vi "PID water height and temperature.vi"(4 "State":i16, 5 "Time":dbl format="%.2f", 6 "Sensor Values":dbl[](array[numeric]), 7 "Set Points":dbl[](array[numeric])) -> (0 "required data":T1={"Set Point names"=["cold/hot output (0/1)", "valve on time (s)", "T target (C)", "H min (cm)", "H abort fill (cm)", "P Kc", "I Ti (s)", "D Td (s)"], "required number of setpoints"=8, "required number of sensors"=2, "Sensor names"=["temperature (C)", "water depth (cm)"]}, 3 "output value":dbl)   [LabVIEW 2019]
uses:
  <vilib>/addons/control/pid/pid.llb/PID (DBL).vi
  <vilib>/addons/control/pid/NI_PID_pid.lvlib
panel:
  out "PID":dbl
  out "Enum 2":enum16{"Waiting", "Filling"}(ring)
  # "Enter the correct information for this control code in the required data structure below. Then make the current value default by right clicking on the border of the data structure."
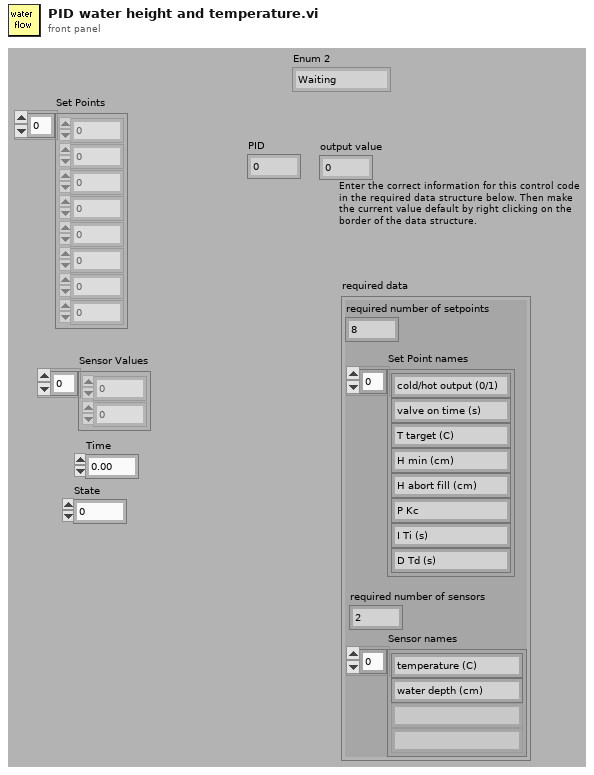
[diagram p1: front panel]
types:
  T1 = cluster{"Set Point names":string[], "required number of setpoints":u8, "required number of sensors":u8, "Sensor names":string[]}
  T2 = cluster{"Set Points[0]":dbl, "Set Points[1]":dbl, "Set Points[2]":dbl, "Set Points[3]":dbl, "Set Points[4]":dbl, "Set Points[5]":dbl, "Set Points[6]":dbl, "Set Points[7]":dbl}
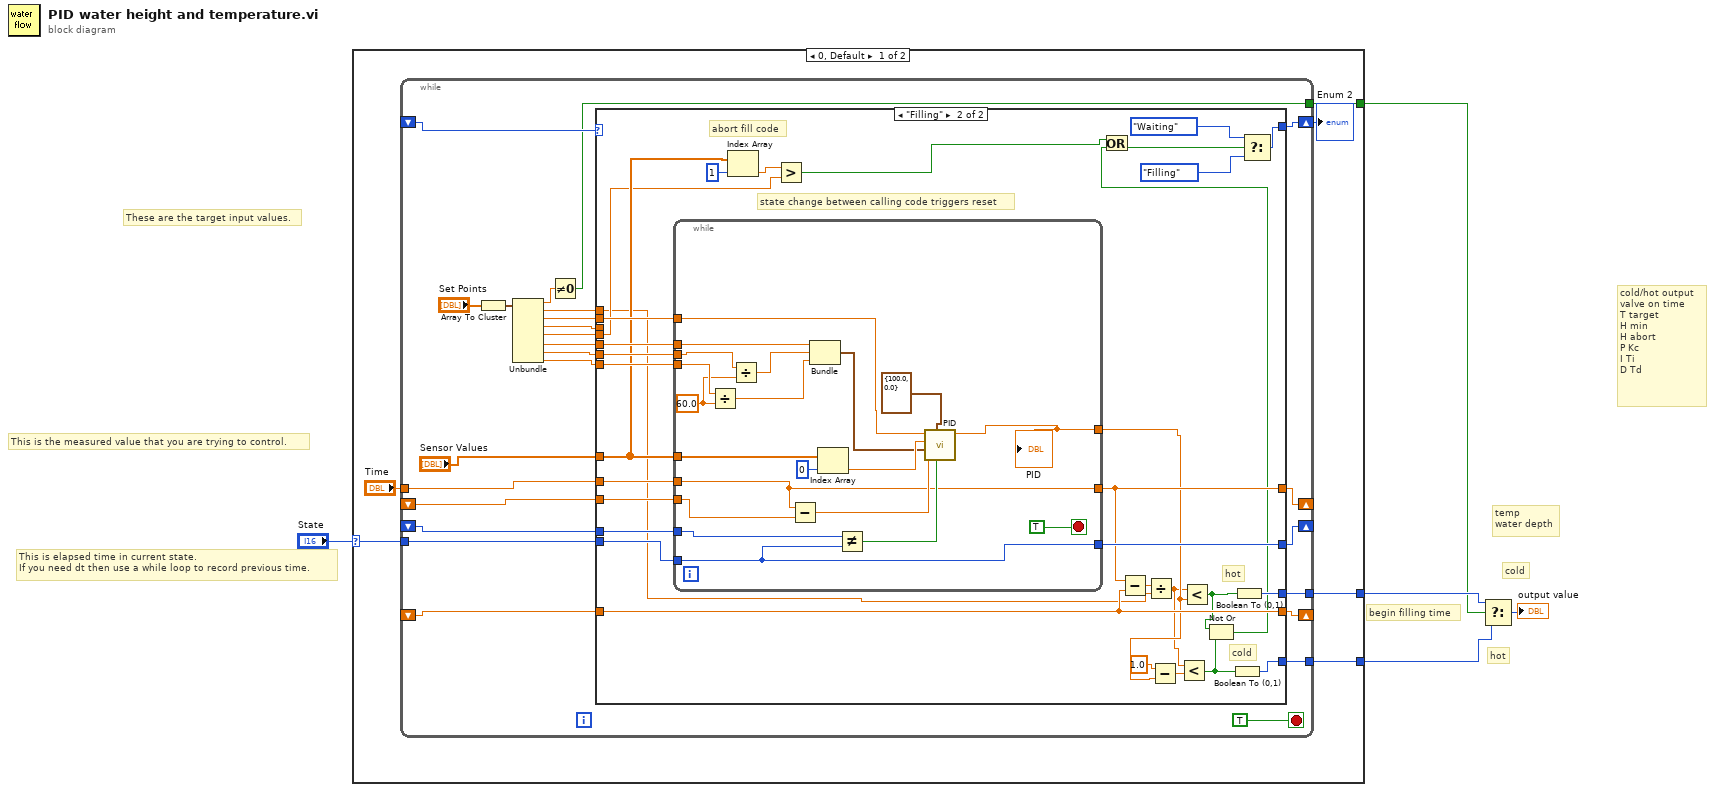
[diagram p0: block diagram]
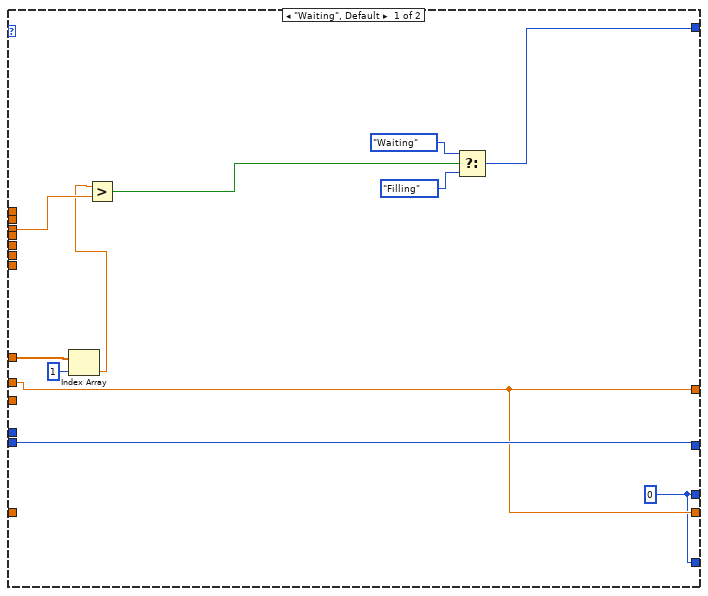
[diagram p2: hidden frame]
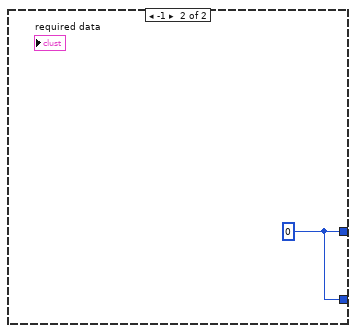
[diagram p3: hidden frame]
diagram:
  # "begin filling time"
  # "hot"
  # "cold"
  # "temp\nwater depth"
  # "cold/hot output\nvalve on time\nT target\nH min\nH abort\nP Kc\nI Ti\nD Td"
  # "These are the target input values."
  # "This is the measured value that you are trying to control."
  # "This is elapsed time in current state.\nIf you need dt then use a while loop to record previous time."
  n1 = case shown="0, Default" "State" {
    selector: "State" -> [w11 _]
    tunnel: [w9 _] -> w2
    tunnel: [w8 w99] -> w3
    tunnel: [w7 w99] -> w1
    frame 0, Default {
      n2 = while {
        tunnel: w11 -> [w36]
        shift-right: [w34] -> w6
        shift-left: _ -> [w24]
        shift-right: [w21] -> _
        shift-left: _ -> [w22]
        shift-right: [w18] -> _
        shift-left: _ -> [w20]
        tunnel: "Time" -> [w19]
        tunnel: [w16] -> w9
        shift-right: [w15] -> _
        shift-left: _ -> [w14]
        tunnel: [w13] -> w8
        tunnel: [w12] -> w7
        stop <- TRUE stop-if-true
        n3 = Array To Cluster(array="Set Points") -> (cluster=w32:T2)
        n4 = Unbundle(w32) -> ("Set Points[0]"=w17:dbl, "Set Points[1]"=w26:dbl, "Set Points[2]"=w27:dbl, "Set Points[3]"=w25:dbl, "Set Points[4]"=w23:dbl, "Set Points[5]"=w30:dbl, "Set Points[6]"=w29:dbl, "Set Points[7]"=w28:dbl)
        n5 = Not Equal To 0?(x=w17) -> (x != 0?=w16:bool)
        n6 = case shown="\"Filling\"" w24 {
          tunnel: w36 -> [w39 w78]
          tunnel: [w45 w70] -> w34
          tunnel: "Sensor Values" -> [w43 w68]
          tunnel: w30 -> [_ w77]
          tunnel: w29 -> [_ w76]
          tunnel: w28 -> [_ w75]
          tunnel: w27 -> [_ w74]
          tunnel: w26 -> [_ w59]
          tunnel: w25 -> [w42 _]
          tunnel: w20 -> [_ w73]
          tunnel: w23 -> [_ w66]
          tunnel: w22 -> [_ w65]
          tunnel: [w39 w64] -> w21
          tunnel: w19 -> [w38 w63]
          tunnel: [w38 w62] -> w18
          tunnel: [w38 w61] -> w15
          tunnel: w14 -> [_ w61]
          tunnel: [w37 w54] -> w13
          tunnel: [w37 w53] -> w12
          frame "Waiting", Default {
            w37 = i16 0
            n7 = Index Array(array=w43, index=1) -> (element=w41:dbl)
            n8 = Greater?(x=w41, y=w42) -> (0:w40:bool)
            n9 = Select(t=enum16{"Waiting", "Filling"}."Waiting" ("Enum"), s=w40, f=enum16{"Waiting", "Filling"}."Filling" ("Enum")) -> (s? t:f=w45:enum16{"Waiting", "Filling"})
          }
          frame "Filling" {
            # "cold"
            # "hot"
            # "abort fill code"
            # "state change between calling code triggers reset"
            n10 = while {
              tunnel: [w84] -> w57
              tunnel: w78 -> [w87]
              tunnel: w68 -> [w91]
              tunnel: w77 -> [w90]
              tunnel: w76 -> [w81]
              tunnel: w75 -> [w83]
              tunnel: w74 -> [w89]
              tunnel: w73 -> [w86]
              tunnel: w65 -> [w88]
              tunnel: [w87] -> w64
              tunnel: w63 -> [w85]
              tunnel: [w85] -> w62
              stop <- TRUE stop-if-true
              w79 = 60.0 ("y")
              n11 = Divide(x=w83, y=w79) -> (x/y=w82:dbl)
              n12 = Divide(x=w81, y=w79) -> (x/y=w80:dbl)
              n13 = Subtract(x=w85, y=w86) -> (x-y=w97:dbl)
              n14 = Bundle("Set Points[5]"=w90, w80, w82) -> (w93:cluster{"Set Points[5]":dbl, dbl, dbl})  [unwired: 1 in]
              n15 = Index Array(array=w91, index=0) -> (element=w95:dbl)
              n16 = Not Equal?(x=w88, y=w87) -> (x != y?=w94:bool)
              n17 = call-poly <vilib>:"PID.vi"("reinitialize? (F)"=w94, "output range"=cluster{"output high":dbl, "output low":dbl} {"output high"=100.0, "output low"=0.0}, "dt (s)"=w97, "PID gains"=w93, "process variable"=w95, "setpoint"=w89) -> ("output"=w84:dbl)  [unwired: 4 in, 1 out]
              "PID" <- w84
            }
            n18 = Index Array(array=w68, index=1) -> (element=w67:dbl)
            n19 = Greater?(x=w67, y=w66) -> (0:w49:bool)
            n20 = Subtract(x=w62, y=w61) -> (x-y=w60:dbl)
            n21 = Divide(x=w60, y=w59) -> (x/y=w56:dbl)
            n22 = Subtract(x=1.0, y=w57) -> (x-y=w55:dbl)
            n23 = Less?(x=w56, y=w55) -> (x < y?=w51:bool)
            n24 = Less?(x=w56, y=w57) -> (x < y?=w52:bool)
            n25 = Not Or(1:w51, 2:w52) -> (0:w48:bool)
            n26 = Or(x=w49, y=w48) -> (x .or. y?=w50:bool)
            n27 = Boolean To (0,1)(Boolean=w51) -> (0, 1=w53:i16)
            n28 = Boolean To (0,1)(Boolean=w52) -> (0, 1=w54:i16)
            n29 = Select(t=enum16{"Waiting", "Filling"}."Waiting" ("Enum"), s=w50, f=enum16{"Waiting", "Filling"}."Filling" ("Enum")) -> (s? t:f=w70:enum16{"Waiting", "Filling"})
          }
        }
      }
      "Enum 2" <- w6
    }
    frame -1 {
      w99 = i16 0
    }
  }
  n30 = Select(t=w3, s=w2, f=w1) -> (s? t:f=→"output value":i16)
